vi "d(f4+g4u)_dx4.vi"(2 "x3_":dbl, 4 "x4_":dbl) -> (22 "d(f4+g4u)/dx4":dbl)   [LabVIEW 2014]
uses:
  <vilib>/Simulation/Implementation/Shared/SIMSCR Execution Mode.ctl
  <vilib>/Simulation/Scripting/Companion Diagram/SimConfigNode/SimParams.ctl
  <vilib>/Simulation/Scripting/Companion Diagram/SimConfigNode/_simSolvers.ctl
  <vilib>/Simulation/Param Hierarchy/Typedefs/SIMPH Param Control Actions.ctl
  <vilib>/Simulation/Implementation/Shared/NILVSim_ParamChanged.vi
  <vilib>/Simulation/Implementation/Shared/NILVSIM_BeginStep.vi
  <vilib>/Simulation/Implementation/Shared/NILVSim_Manager.vi
  <vilib>/Utility/error.llb/Clear Errors.vi
  <vilib>/Simulation/Implementation/Shared/NILVSim_FinalizeModel.vi
  <vilib>/Simulation/Implementation/Shared/SIM Unbundle Sim Info.vi
  <vilib>/Simulation/Implementation/Shared/SIMSH Read Queue.vi
  <vilib>/Simulation/Implementation/Shared/NILVSim_Initialize.vi
  <vilib>/Simulation/Utility/Implementation/NILVSim Get Time and IsAcceptedStep.vi
  <vilib>/Simulation/Implementation/Shared/NILVSim_GetModelError.vi
  <vilib>/Simulation/Implementation/Shared/SIM SimErrorHandler.vi
  <vilib>/Simulation/Implementation/Shared/SIM Bundle Sim Info.vi
  <vilib>/Simulation/Scripting/Companion Diagram/SimConfigNode/SimDog.xnode
  <vilib>/Simulation/Implementation/XNodeFramework/SimXNode/SimX.xnode
  <vilib>/Simulation/Implementation/Shared/NI_SIM_Implementation.lvlib
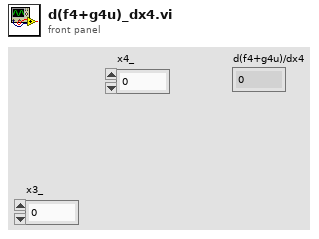
[diagram p1: front panel]
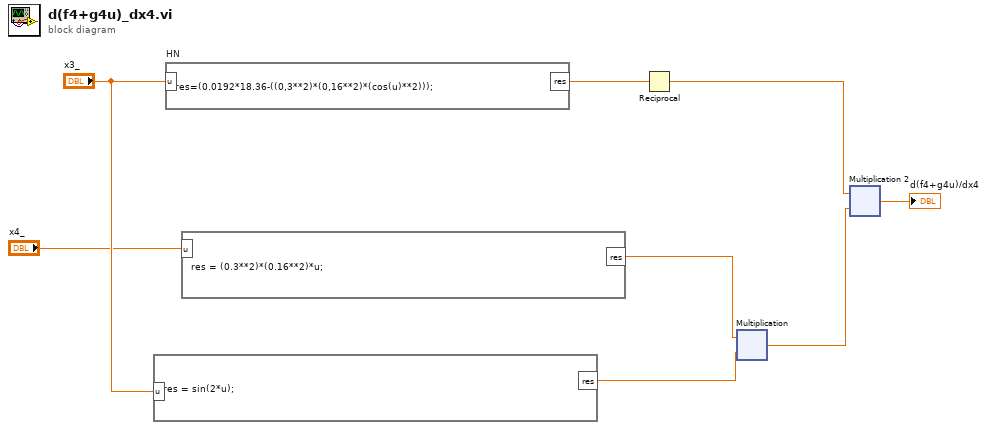
[diagram p0: block diagram]
diagram:
  n1 = formula code="res = sin(2*u);" ("Formelknoten 2")("u"="x3_") -> ("res"=w5:dbl)
  n2 = formula code="res=(0.0192*18.36-((0,3**2)*(0,16**2)*(cos(u)**2)));" "HN"("u"="x3_") -> ("res"=w8:dbl)
  n3 = formula code="res = (0.3**2)*(0.16**2)*u;" ("Formelknoten")("u"="x4_") -> ("res"=w4:dbl)
  n4 = Reciprocal ("Math\\nFunction")(x=w8) -> (1/x=w2:dbl)
  n5 = xnode ("Multiplication")("Operand1"=w4, "Operand2"=w5) -> ("Result"=w6:dbl)
  n6 = xnode ("Multiplication 2")("Operand1"=w2, "Operand2"=w6) -> ("Result"=→"d(f4+g4u)/dx4":dbl)
